vi "FRA_UDP_get_time.vi"() -> (1 "epoch time":u32, 3 "array":u8[](array[numeric]))   [LabVIEW 2013]
doc: "formats time to put into first 4 bytes of UDP packet\nepoch time\nbyte array is little endian epoch time of 4 bytes\nLabview time to epoch time conversion"
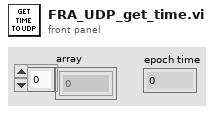
[diagram p1: front panel]
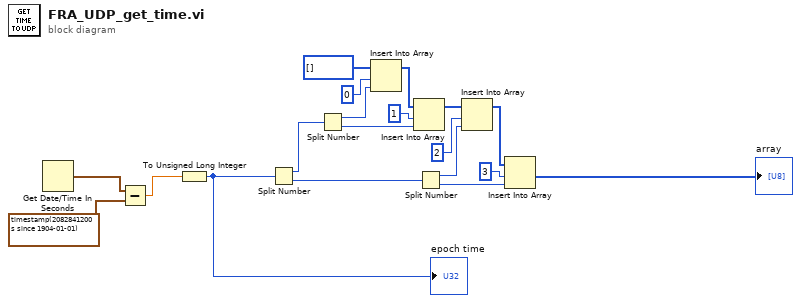
[diagram p0: block diagram]
diagram:
  n1 = Get Date/Time In Seconds() -> (seconds since 1Jan1904=w17:timestamp)
  n2 = Subtract(x=w17, y=timestamp(2082841200 s since 1904-01-01) ("current time")) -> (x-y=w19:dbl)
  n3 = To Unsigned Long Integer(number=w19) -> (unsigned 32bit integer=w16:u32)
  "epoch time" <- w16
  n4 = Split Number(x=w16) -> (hi(x)=w2:u16, lo(x)=w1:u16)
  n5 = Split Number(x=w2) -> (hi(x)=w4:u8, lo(x)=w9:u8)
  n6 = Insert Into Array(array=u8[] [], index=0, new element=w4) -> (w12:u8[])
  n7 = Insert Into Array(array=w12, index=1, new element=w9) -> (w13:u8[])
  n8 = Split Number(x=w1) -> (hi(x)=w10:u8, lo(x)=w11:u8)
  n9 = Insert Into Array(array=w13, index=2, new element=w10) -> (w14:u8[])
  n10 = Insert Into Array(array=w14, index=3, new element=w11) -> (→"array":u8[])
